vi "Update FP.vi"(6 "subpanel to main command event":T2, 7 "defer fp updates (T)":bool=TRUE, 8 "error in (no error)":errorcluster, 10 "fp refs":T1, 11 "steering frame ref in":refnum<data-value>) -> (0 "error out":errorcluster, 3 "steering frame ref out":refnum<data-value>)   [LabVIEW 2017, in "NI_Robotics_Configure Steering Frame.lvlib" / "Ackermann Frame Subpanel.lvlib"]
uses:
  <vilib>/robotics/Dialog/Configure Steering Frame/Ackermann Frame Subpanel/Ackermann Frame Subpanel.lvlib
  <vilib>/robotics/Steering/Ackermann Steering Frame/NI_Robotics_Ackermann Steering Frame.lvclass
  c:/Program Files (x86)/National Instruments/LabVIEW 2017/vi.lib/robotics/Steering/Steering Frame/NI_Robotics_Steering Frame.lvclass
  <vilib>/robotics/Dialog/Configure Steering Frame/Subpanel to Main Command Event.ctl
  <vilib>/robotics/Dialog/Configure Steering Frame/Subpanel to Main Command.ctl
  <vilib>/robotics/Dialog/Configure Steering Frame/Ackermann Frame Subpanel/FP Refs.ctl
  <vilib>/robotics/Steering/Ackermann Steering Frame/NI_Robotics_Ackermann Steering Frame.lvclass/NI_Robotics_Ackermann Steering Frame.ctl
  <vilib>/robotics/Steering/Steering Frame/NI_Robotics_Steering Frame.lvclass/NI_Robotics_Steering Frame.ctl
  <vilib>/robotics/Steering/Steering Frame/Get Single Wheel in Steering Frame.vi
  <vilib>/robotics/Steering/Steering Frame/Get Multiple Wheels in Steering Frame.vi
  <vilib>/robotics/Steering/Wheel/Get Fixed Wheel Information.vi
  <vilib>/robotics/Steering/Wheel/NI_Robotics_Wheel.lvclass
  <vilib>/robotics/Steering/Steering Frame/NI_Robotics_Steering Frame.lvclass
  c:/Program Files (x86)/National Instruments/LabVIEW 2017/vi.lib/robotics/Steering/Special Steering Frame/NI_Robotics_Special Steering Frame.lvclass
  <vilib>/robotics/Dialog/Configure Steering Frame/NI_Robotics_Configure Steering Frame.lvlib
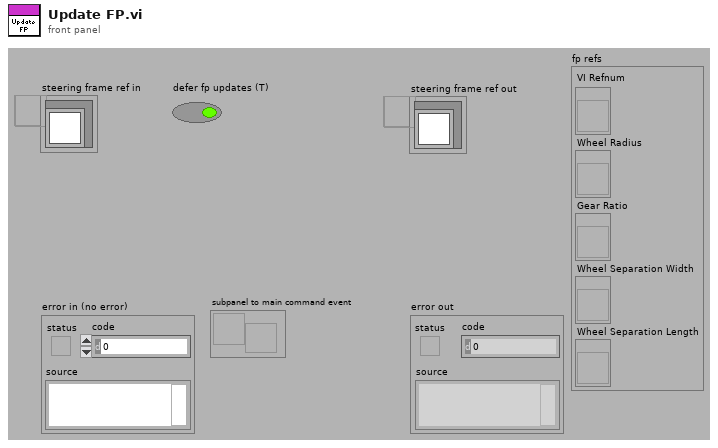
[diagram p1: front panel]
types:
  T1 = typedef "NI_Robotics_Configure Steering Frame.lvlib/Ackermann Frame Subpanel.lvlib/FP Refs.ctl" = cluster{"VI Refnum":refnum<vi>, "Wheel Radius":refnum<vi>, "Gear Ratio":refnum<vi>, "Wheel Separation Width":refnum<vi>, "Wheel Separation Length":refnum<vi>}
  T2 = typedef "NI_Robotics_Configure Steering Frame.lvlib/Subpanel to Main Command Event.ctl" = refnum<user-event>
  T3 = typedef "NI_Robotics_Wheel.lvclass/Wheel Parameters.ctl" = cluster{"wheel radius":dbl, "gear ratio":dbl, "forward rotation direction":T4}
  T4 = typedef "NI_Robotics_Wheel.lvclass/Rotation Direction.ctl" = u16
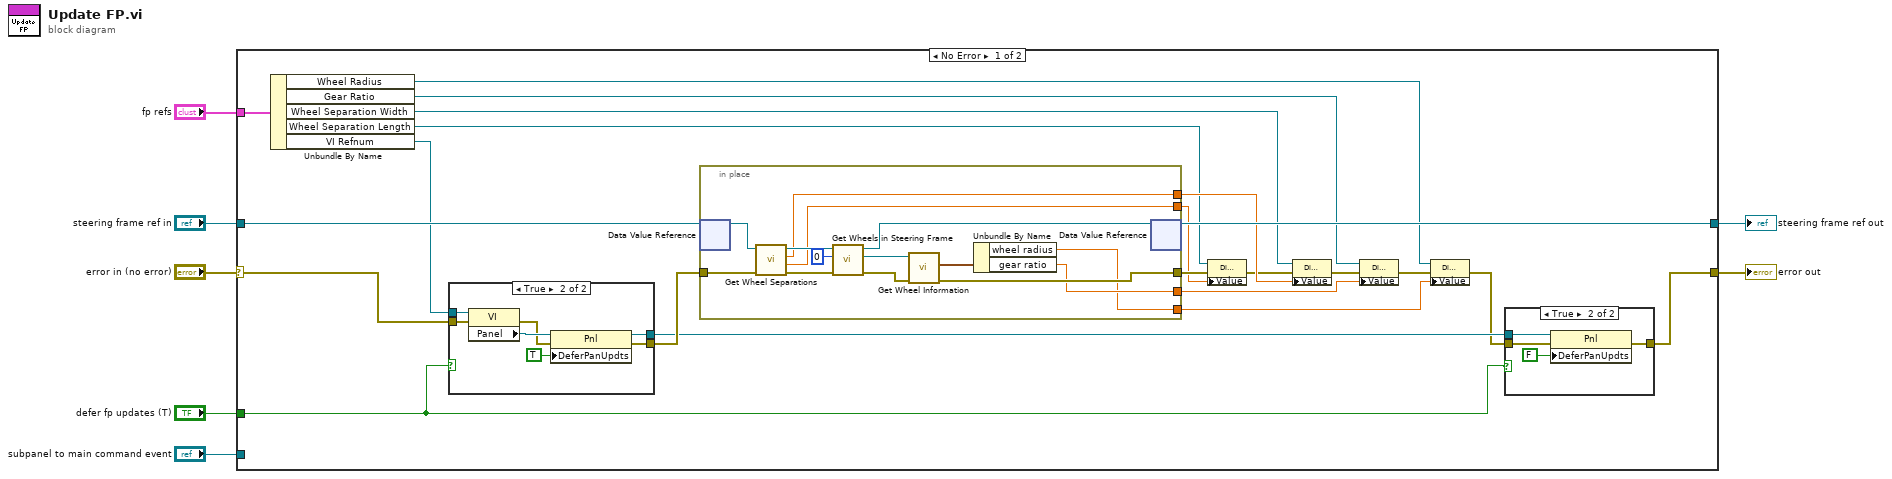
[diagram p0: block diagram]
diagram:
  n1 = case shown="No Error" "error in (no error)" {
    selector: "error in (no error)" -> [w26 w57]
    tunnel: "steering frame ref in" -> [w29 w58]
    tunnel: [w28 w58] -> w5
    tunnel: [w23 w57] -> w4
    tunnel: "subpanel to main command event" -> [_ _]
    tunnel: "fp refs" -> [w27 _]
    tunnel: "defer fp updates (T)" -> [w22 _]
    frame No Error {
      n2 = Unbundle By Name(w27) -> ("Wheel Radius"=w15:refnum<vi>, "Gear Ratio"=w17:refnum<vi>, "Wheel Separation Width"=w20:refnum<vi>, "Wheel Separation Length"=w11:refnum<vi>, "VI Refnum"=w12:refnum<vi>)
      n3 = case shown="True" w22 {
        tunnel: [_ w40] -> w24
        tunnel: w12 -> [_ w39]
        tunnel: w26 -> [w35 w38]
        tunnel: [w35 w36] -> w25
        frame False {
        }
        frame True {
          n4 = property class="VI"(reference=w39, error in=w38) -> (error out=w37:errorcluster, "Panel"=w42:refnum<vi>)  [unwired: 1 out]
          n5 = property class="Pnl"(reference=w42, error in=w37, "DeferPanUpdts"=TRUE ("Defer Panel Updates")) -> (reference out=w40:refnum<vi>, error out=w36:errorcluster)
        }
      }
      n6 = in-place {
        in-place-border: w25 -> [w45]
        in-place-border: [w52] -> w9
        in-place-border: [w46] -> w21
        in-place-border: [w50] -> w16
        in-place-border: [w49] -> w14
        in-place-border: [w43] -> w8
        n7 = in-place-dvr #1(w29) -> (w48:refnum<class "NI_Robotics_Ackermann Steering Frame.lvclass">)  [unwired: 1 out]
        n8 = call <vilib>:"Get Wheel Separations.vi"("error in (no error)"=w45, "ackermann steering frame in"=w48) -> ("error out"=w44:errorcluster, "wheel separation length"=w43:dbl, "wheel separation width"=w46:dbl, "ackermann steering frame out"=w47:refnum<class "NI_Robotics_Ackermann Steering Frame.lvclass">)  [unwired: 6 in]
        n9 = call-poly <vilib>:"Get Wheels in Steering Frame.vi"("error in (no error)"=w44, "wheel index"=0, "steering frame in"=w47) -> ("error out"=w53:errorcluster, "wheel"=w54:refnum<class "NI_Robotics_Wheel.lvclass">, "steering frame out"=w55:refnum<class "NI_Robotics_Ackermann Steering Frame.lvclass">)  [unwired: 2 in, 4 out]
        n10 = call-poly <vilib>:"Get Wheel Information.vi"("error in (no error)"=w53, "wheel in"=w54) -> ("error out"=w52:errorcluster, "wheel parameters"=w51:T3)  [unwired: 5 in, 3 out]
        n11 = Unbundle By Name(w51) -> ("wheel radius"=w49:dbl, "gear ratio"=w50:dbl)
        n12 = in-place-dvr #1(w55) -> (w28:refnum<data-value>)  [unwired: 1 out]
      }
      n13 = property class="DigNum (strict)"(reference=w11, error in=w9, "Value"=w8) -> (error out=w10:errorcluster)  [unwired: 1 out]
      n14 = property class="DigNum (strict)"(reference=w20, error in=w10, "Value"=w21) -> (error out=w19:errorcluster)  [unwired: 1 out]
      n15 = property class="DigNum (strict)"(reference=w17, error in=w19, "Value"=w16) -> (error out=w18:errorcluster)  [unwired: 1 out]
      n16 = property class="DigNum (strict)"(reference=w15, error in=w18, "Value"=w14) -> (error out=w13:errorcluster)  [unwired: 1 out]
      n17 = case shown="True" w22 {
        tunnel: w24 -> [_ w33]
        tunnel: w13 -> [w30 w32]
        tunnel: [w30 w31] -> w23
        frame False {
        }
        frame True {
          n18 = property class="Pnl"(reference=w33, error in=w32, "DeferPanUpdts"=FALSE ("Defer Panel Updates")) -> (error out=w31:errorcluster)  [unwired: 1 out]
        }
      }
    }
    frame Error {
    }
  }
  "steering frame ref out" <- w5
  "error out" <- w4
